vi "emi_SMLoop Get State.vi"   [LabVIEW 2011]
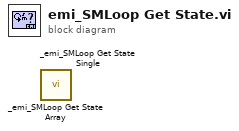
[diagram p0: block diagram]
diagram:
  n1 = call "_emi_SMLoop Get State Array.vi"() -> ()  [unwired: 9 in, 7 out]
  n2 = call "_emi_SMLoop Get State Single.vi"() -> ()  [unwired: 9 in, 7 out]
